vi "Write Tag-ID Map.vi"(8 "error in (no error)":errorcluster, 10 "Tag-ID Map":map{string, i64}(c390), 11 "Node Actor in":refnum<class "Node Actor.lvclass">) -> (0 "error out":errorcluster, 3 "Node Actor out":refnum<class "Node Actor.lvclass">)   [LabVIEW 2024, in "Node Actor.lvclass"]
uses:
  Node Actor.lvclass
  Node Actor.lvclass/Node Actor.ctl
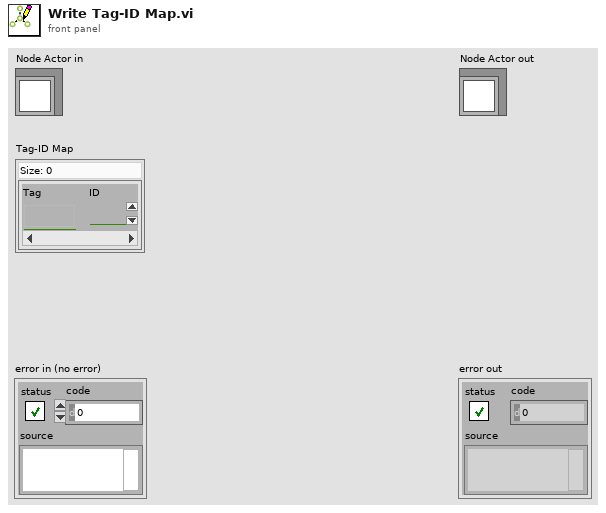
[diagram p1: front panel]
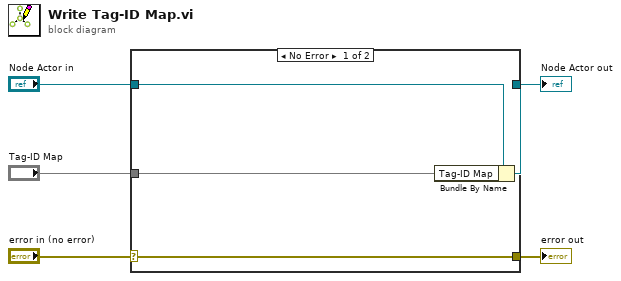
[diagram p0: block diagram]
diagram:
  n1 = case shown="No Error" "error in (no error)" {
    selector: "error in (no error)" -> [w9 w10]
    tunnel: [w9 w10] -> w4
    tunnel: [w7 w11] -> w2
    tunnel: "Node Actor in" -> [w8 w11]
    tunnel: "Tag-ID Map" -> [w6 _]
    frame No Error {
      n2 = Bundle By Name(cluster=w8, "Tag-ID Map"=w6) -> (w7:refnum<class "Node Actor.lvclass">)
    }
    frame Error {
    }
  }
  "error out" <- w4
  "Node Actor out" <- w2
